vi "CLT_5PtCalStateMach.vi"(7 "Full Cfg":T4, 8 "Index In":i32, 10 "Pump Signals":T8, 11 "Cal State In":T1) -> (0 "Index Out":i32, 2 "Pump Cmds":T2, 3 "Cal State Out":T1)   [LabVIEW 2024]
doc: "The \"Run Test\" button selects between MANUAL adjustment of Set Point (SP) by the user or AUTO mode, where:\n1. Start, initial state drains until the tank is empty\n2. Filling, Auto set of SP to Max Fill Inches (or recipie)\n3. FULL Pause when full\n4. Draining Auto set of SP to 0 (or recipie)\n5. EMPTY Paue when empty\n6. Done SP set to 0."
uses:
  Control Definitions/Def_PumpSignals.ctl
  Control Definitions/Def FullCfg.ctl
  Control Definitions/Def BenchCfg.ctl
  Control Definitions/Def PumpCtlRefs.ctl
  Control Definitions/Def_PumpSpeed.ctl
  Control Definitions/Def Bench Status.ctl
  Control Definitions/Def_PumpCmds.ctl
  Control Definitions/DEF_5ptCalState.ctl
  Control Definitions/Global 2.vi
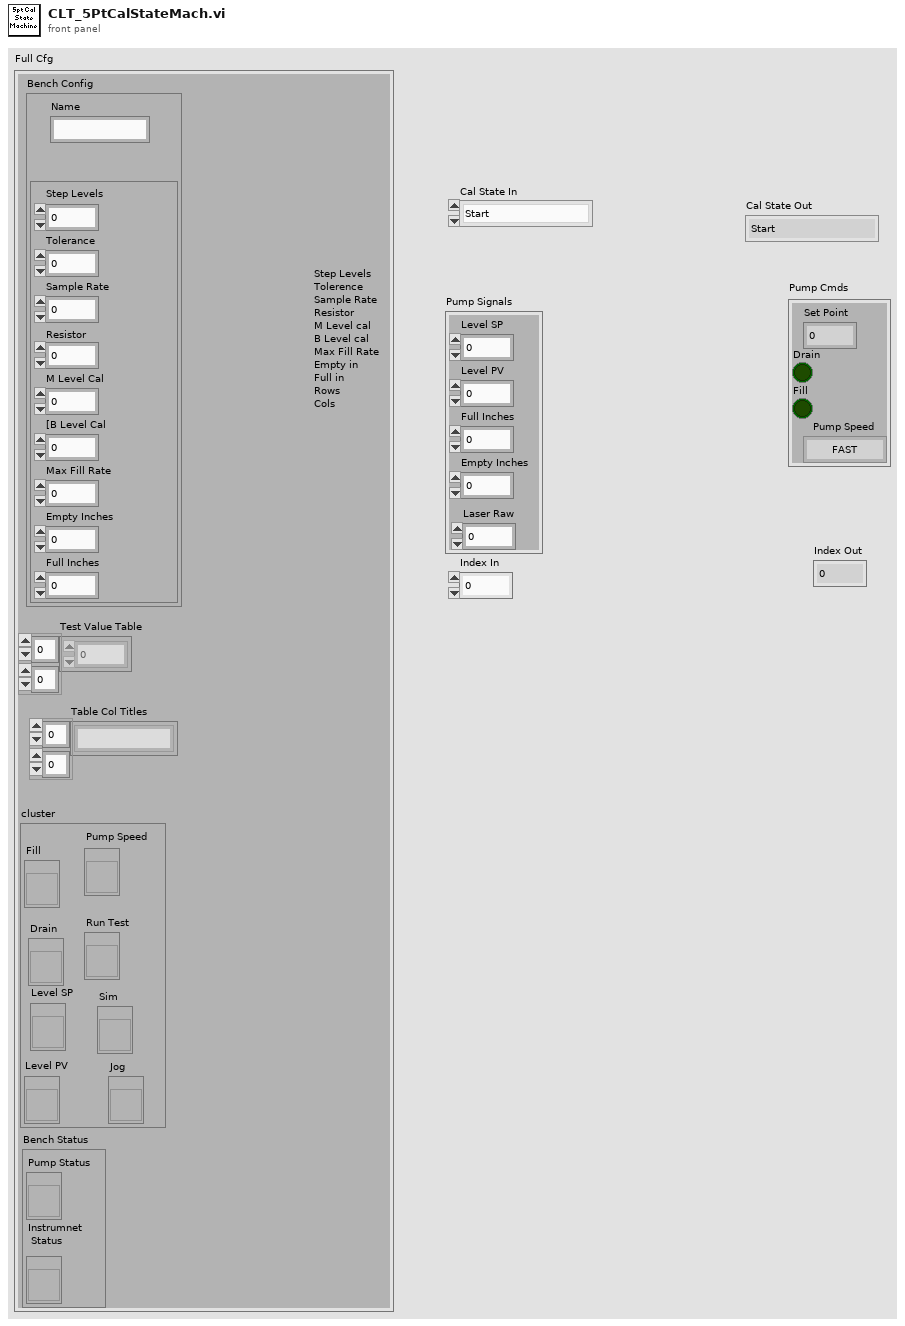
[diagram p1: front panel]
types:
  T1 = typedef "DEF_5ptCalState.ctl" = enum16{"Start", "Load Tester", "Go Auto", "Level 1", "Reveiw ", "Save", "Exit"}
  T2 = typedef "Def_PumpCmds.ctl" = cluster{"Set Point":dbl, "Drain":bool, "Fill":bool, "Pump Speed ":T3}
  T3 = typedef "Def_PumpSpeed.ctl" = enum16{"FAST", "SLOW", "CREEP", "STOP"}
  T4 = typedef "Def FullCfg.ctl" = cluster{"Bench Config":T5, "Test Value Table ":dbl[][], "Table Col Titles":string[][], "cluster":T6, "Bench Status":T7}
  T5 = typedef "Def BenchCfg.ctl" = cluster{"Name":string, cluster{"Step Levels":dbl, "Tolerance":dbl, "Sample Rate":dbl, "Resistor":dbl, "M Level Cal":dbl, "[B Level Cal":dbl, "Max Fill Rate":dbl, "Empty Inches":dbl, "Full Inches":dbl}}
  T6 = typedef "Def PumpCtlRefs.ctl" = cluster{"Fill ":refnum<vi>, "Drain":refnum<vi>, "Level PV":refnum<vi>, "Pump Speed":refnum<vi>, "Run Test":refnum<vi>, "Sim":refnum<vi>, "Jog":refnum<vi>, "Level SP":refnum<vi>}
  T7 = typedef "Def Bench Status.ctl" = cluster{"Pump Status":refnum<vi>, "Instrumnet\n Status":refnum<vi>}
  T8 = typedef "Def_PumpSignals.ctl" = cluster{"Level SP":dbl, "Level PV":dbl, "Full Inches":dbl, "Empty Inches":dbl, "Laser Raw":dbl}
  T9 = cluster{"Level SP":dbl, "X>Pos":bool, "X>Pos":bool, "Pump Speed Out":T3}
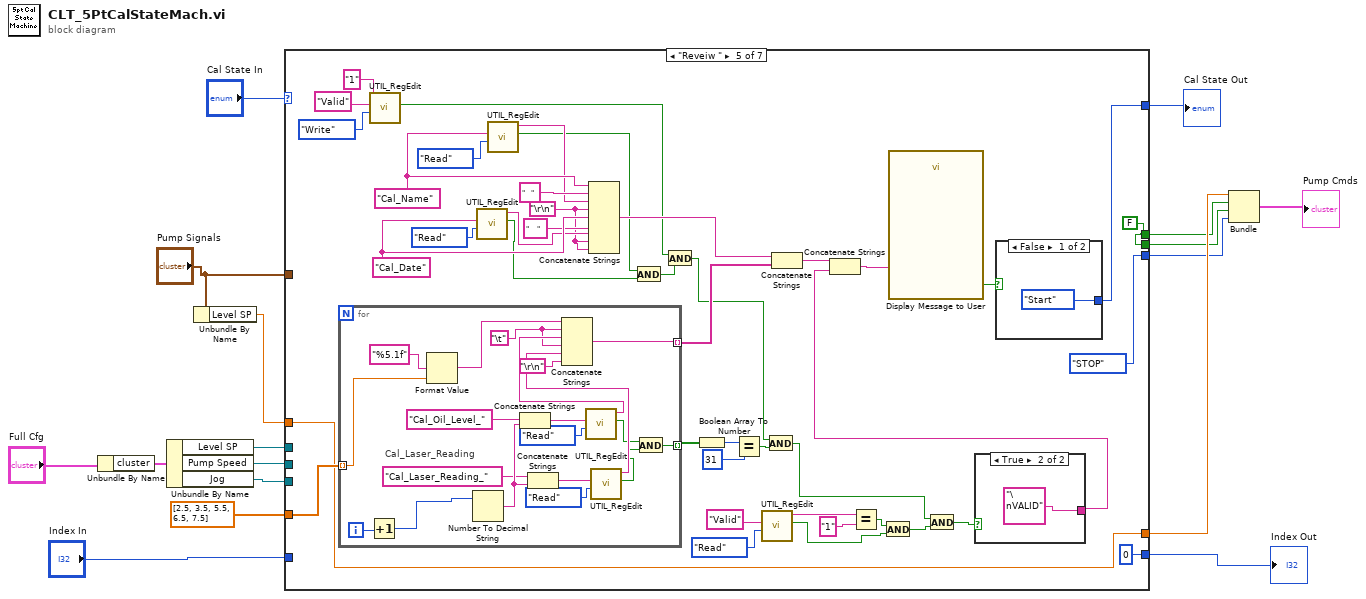
[diagram p0: block diagram]
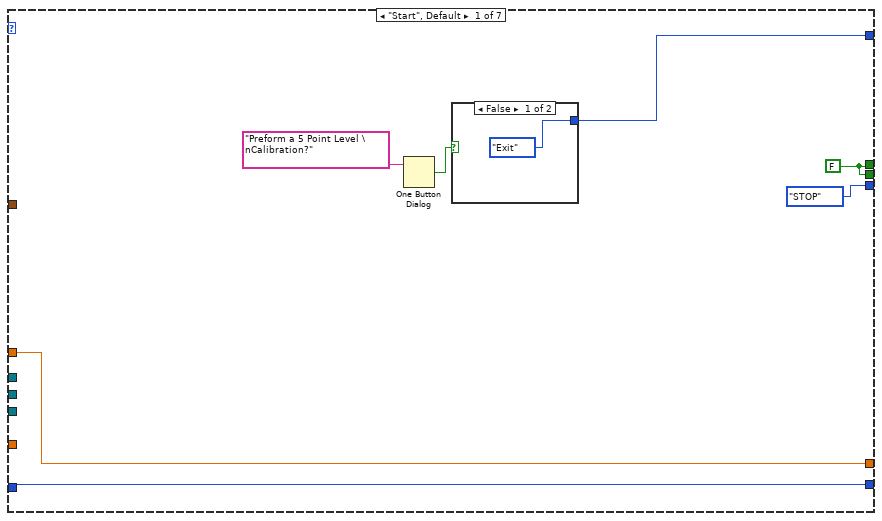
[diagram p2: hidden frame]
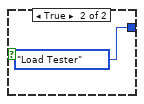
[diagram p3: hidden frame]
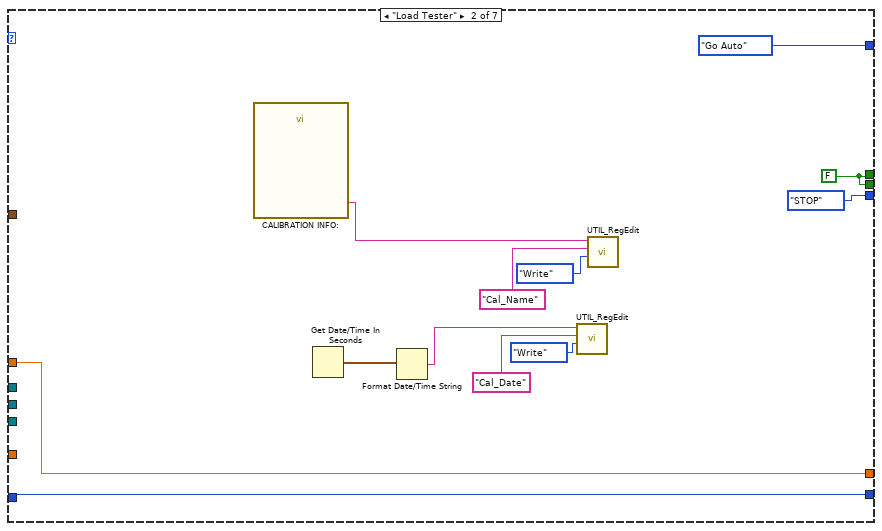
[diagram p4: hidden frame]
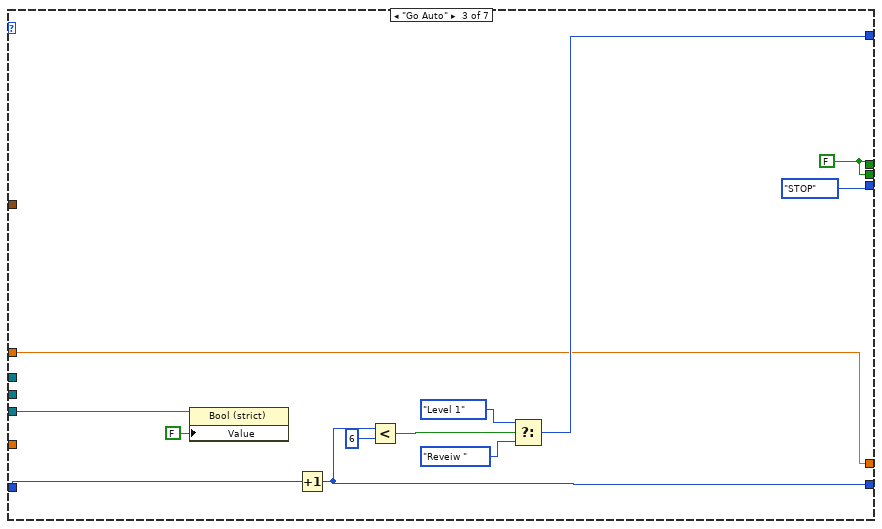
[diagram p5: hidden frame]
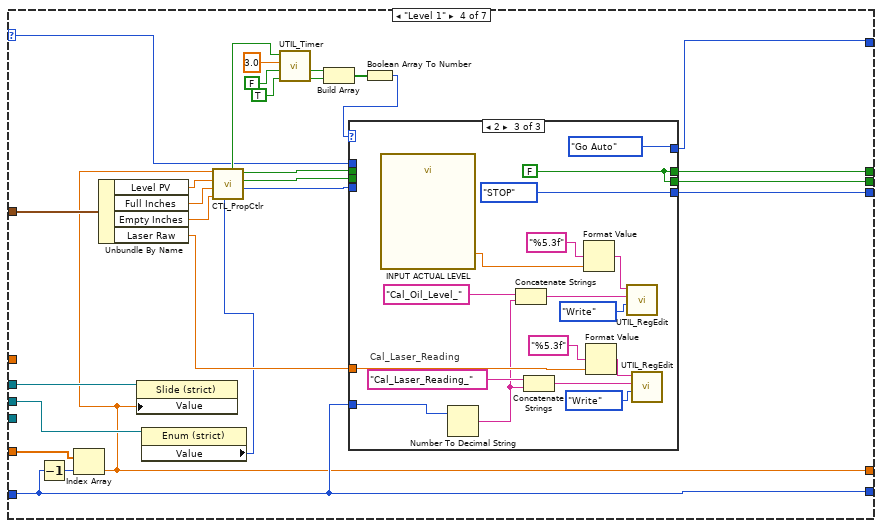
[diagram p6: hidden frame]
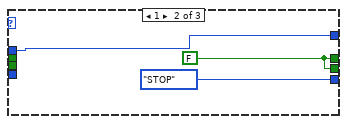
[diagram p8: hidden frame]
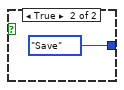
[diagram p9: hidden frame]
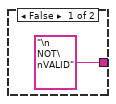
[diagram p10: hidden frame]
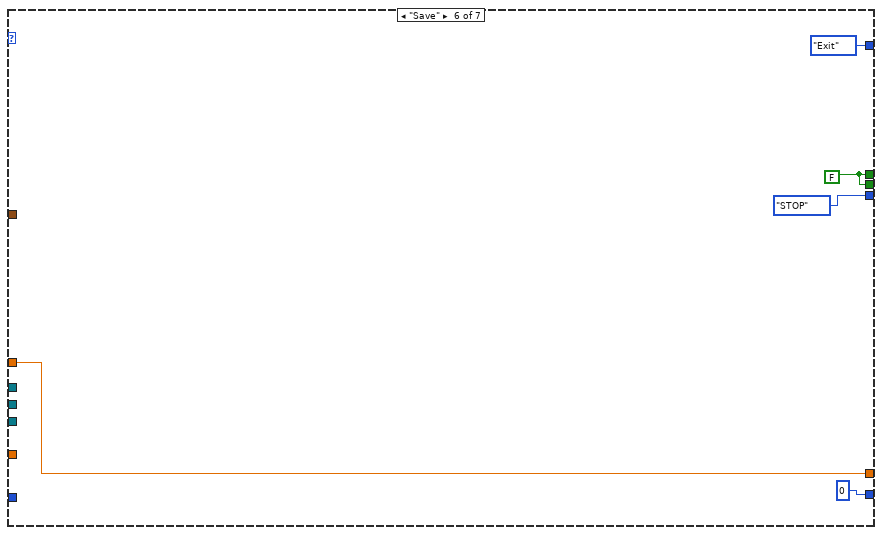
[diagram p11: hidden frame]
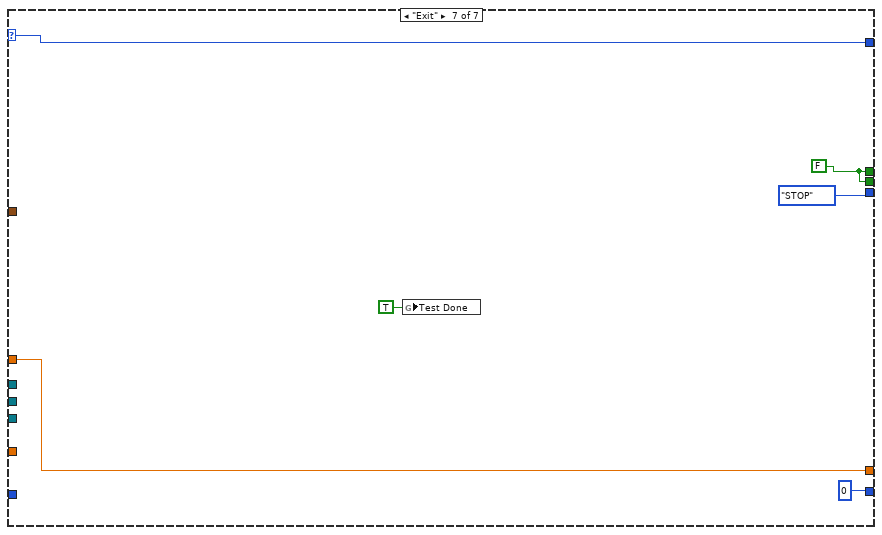
[diagram p12: hidden frame]
diagram:
  n1 = Unbundle By Name("Full Cfg") -> ("cluster"=w16:T6)
  n2 = Unbundle By Name(w16) -> ("Level SP"=w12:refnum<vi>, "Pump Speed"=w13:refnum<vi>, "Jog"=w11:refnum<vi>)
  n3 = Unbundle By Name("Pump Signals") -> ("Level SP"=w3:dbl)
  n4 = case shown="\"Reveiw \"" "Cal State In" {
    selector: "Cal State In" -> [_ _ _ w66 _ _ w175]
    tunnel: [w22 DEF_5ptCalState."Go Auto" w47 w67 w113 DEF_5ptCalState."Exit" ("Cal State In") w175] -> w14
    tunnel: "Pump Signals" -> [_ _ _ w65 _ _ _]
    tunnel: w13 -> [_ _ _ w60 _ _ _]
    tunnel: w12 -> [_ _ _ w58 _ _ _]
    tunnel: w11 -> [_ _ w50 _ _ _ _]
    tunnel: [w21 w30 w46 w55 0 0 0] -> w1
    tunnel: "Index In" -> [w21 w30 w48 w55 _ _ _]
    tunnel: dbl[] [2.5, 3.5, 5.5, 6.5, 7.5] ("Array") -> [_ _ _ w56 w135 _ _]
    tunnel: [w18 w27 w39 w51 w109 w170 w177] -> w9
    tunnel: [w20 w28 w40 w54 w111 w171 w178] -> w8
    tunnel: [w20 w28 w40 w53 w111 w171 w178] -> w7
    tunnel: [Def_PumpSpeed."STOP" ("Pump Speed Out") Def_PumpSpeed."STOP" ("Pump Speed Out") Def_PumpSpeed."STOP" ("Pump Speed Out") w52 Def_PumpSpeed."STOP" ("Pump Speed Out") Def_PumpSpeed."STOP" ("Pump Speed Out") Def_PumpSpeed."STOP" ("Pump Speed Out")] -> w6
    tunnel: w3 -> [w18 w27 w39 _ w109 w170 w177]
    frame "Start", Default {
      w20 = FALSE ("X>Pos")
      n5 = One Button Dialog(message="Preform a 5 Point Level \nCalibration?") -> (true=w23:bool)  [unwired: 1 in]
      n6 = case shown="False" w23 {
        tunnel: [DEF_5ptCalState."Exit" ("Cal State In") DEF_5ptCalState."Load Tester" ("Cal State In")] -> w22
        frame False {
        }
        frame True {
        }
      }
    }
    frame "Load Tester" {
      w28 = FALSE ("X>Pos")
      n7 = call "CALIBRATION INFO:"() -> ("Name"=w32:string)  [unwired: 17 in, 2 out]
      n8 = Get Date/Time In Seconds() -> (seconds since 1Jan1904=w37:timestamp)
      n9 = Format Date/Time String(seconds (now)=w37) -> (date/time string=w38:string)  [unwired: 2 in]
      n10 = call "UTIL_RegEdit.vi"("Mode"=enum16{"Write", "Read", "Delete"}."Write", "String Name"="Cal_Date", "String Value"=w38) -> ()  [unwired: 7 in, 2 out]
      n11 = call "UTIL_RegEdit.vi"("Mode"=enum16{"Write", "Read", "Delete"}."Write", "String Name"="Cal_Name", "String Value"=w32) -> ()  [unwired: 7 in, 2 out]
    }
    frame "Go Auto" {
      w40 = FALSE ("X>Pos")
      n12 = property class="Bool (strict)"(reference=w50, "Value"=FALSE) -> ()  [unwired: 1 in, 2 out]
      n13 = Increment(x=w48) -> (x+1=w46:i32)
      n14 = Less?(x=w46, y=6) -> (x < y?=w44:bool)
      n15 = Select(t=DEF_5ptCalState."Level 1" ("Cal State In"), s=w44, f=DEF_5ptCalState."Reveiw " ("Cal State In")) -> (s? t:f=w47:T1)
    }
    frame "Level 1" {
      n16 = Decrement(x=w55) -> (x-1=w57:i32)
      n17 = Index Array(array=w56, index=w57) -> (element=w51:dbl)
      n18 = Unbundle By Name(w65) -> ("Level PV"=w64:dbl, "Full Inches"=w63:dbl, "Empty Inches"=w62:dbl, "Laser Raw"=w61:dbl)
      n19 = property class="Slide (strict)"(reference=w58, "Value"=w51) -> ()  [unwired: 1 in, 2 out]
      n20 = property class="Enum (strict)"(reference=w60) -> ("Value"=w59:T3)  [unwired: 1 in, 2 out]
      n21 = call "CTL_PropCtlr.vi"("Pump Speed"=w59, "Empty Inches"=w62, "Full Inches"=w63, "Level PV"=w64, "Level SP"=w51) -> ("Pump Speed Out"=w68:T3, "X< Neg"=w69:bool, "X>Pos"=w71:bool, "Neg <X<Pos"=w75:bool)  [unwired: 3 in]
      n22 = call "UTIL_Timer.vi"("Auto Reset"=TRUE, "Reset"=FALSE, "Time (sec)"=3.0, "Start"=w75) -> ("Timed Out"=w73:bool, "Running"=w74:bool)  [unwired: 2 in, 4 out]
      n23 = Build Array(w74, w73) -> (w72:bool[])
      n24 = Boolean Array To Number(Boolean array=w72) -> (number=w70:u32)
      n25 = case shown="2" w70 {
        tunnel: [w82 w85 w102] -> w54
        tunnel: w71 -> [w82 _ _]
        tunnel: [w81 w85 w102] -> w53
        tunnel: w69 -> [w81 _ _]
        tunnel: [w80 Def_PumpSpeed."STOP" ("Pump Speed Out") Def_PumpSpeed."STOP" ("Pump Speed Out")] -> w52
        tunnel: w68 -> [w80 _ _]
        tunnel: [w79 w83 DEF_5ptCalState."Go Auto" ("Cal State In")] -> w67
        tunnel: w66 -> [w79 w83 _]
        tunnel: w61 -> [_ _ w96]
        tunnel: w55 -> [_ _ w92]
        frame 0, Default {
        }
        frame 1 {
          w85 = FALSE ("X>Pos")
        }
        frame 2 {
          w102 = FALSE ("X>Pos")
          # "Cal_Laser_Reading"
          n26 = call "INPUT ACTUAL LEVEL"() -> ("Level"=w93:dbl)  [unwired: 17 in, 2 out]
          n27 = Number To Decimal String(number=w92) -> (decimal integer string=w88:string)  [unwired: 1 in]
          n28 = Concatenate Strings("Cal_Oil_Level_", w88) -> (w86:string)
          n29 = Concatenate Strings("Cal_Laser_Reading_", w88) -> (w91:string)
          n30 = Format Value(format string="%5.3f", value (0)=w93) -> (output string=w94:string)  [unwired: 1 in]
          n31 = Format Value(format string="%5.3f", value (0)=w96) -> (output string=w100:string)  [unwired: 1 in]
          n32 = call "UTIL_RegEdit.vi"("Mode"=enum16{"Write", "Read", "Delete"}."Write", "String Name"=w86, "String Value"=w94) -> ()  [unwired: 7 in, 2 out]
          n33 = call "UTIL_RegEdit.vi"("Mode"=enum16{"Write", "Read", "Delete"}."Write", "String Name"=w91, "String Value"=w100) -> ()  [unwired: 7 in, 2 out]
        }
      }
    }
    frame "Reveiw " {
      w111 = FALSE ("X>Pos")
      w136 = "\r\n"
      w142 = "Cal_Name"
      w139 = "Cal_Date"
      n34 = for {
        tunnel: w135 -> [w158] mode=indexing
        tunnel: [w152] -> w133 mode=indexing
        tunnel: [w149] -> w132 mode=indexing
        i -> [w161]
        w155 = "\t"
        # "Cal_Laser_Reading"
        n35 = Increment(x=w161) -> (x+1=w160:i32)
        n36 = Format Value(format string="%5.1f", value (0)=w158) -> (output string=w157:string)  [unwired: 1 in]
        n37 = Number To Decimal String(number=w160) -> (decimal integer string=w168:string)  [unwired: 1 in]
        n38 = Concatenate Strings("Cal_Oil_Level_", w168) -> (w167:string)
        n39 = Concatenate Strings("Cal_Laser_Reading_", w168) -> (w166:string)
        n40 = call "UTIL_RegEdit.vi"("Mode"=enum16{"Write", "Read", "Delete"}."Read", "String Name"=w167) -> ("Success?"=w151:bool, "Value Read"=w156:string)  [unwired: 8 in]
        n41 = call "UTIL_RegEdit.vi"("Mode"=enum16{"Write", "Read", "Delete"}."Read", "String Name"=w166) -> ("Success?"=w150:bool, "Value Read"=w154:string)  [unwired: 8 in]
        n42 = Concatenate Strings(w157, w155, w156, w155, w154, "\r\n") -> (w152:string)
        n43 = And(x=w151, y=w150) -> (x .and. y?=w149:bool)
      }
      n44 = call "UTIL_RegEdit.vi"("Mode"=enum16{"Write", "Read", "Delete"}."Write", "String Name"="Valid", "String Value"="1") -> ("Success?"=w103:bool)  [unwired: 7 in, 1 out]
      n45 = call "UTIL_RegEdit.vi"("Mode"=enum16{"Write", "Read", "Delete"}."Read", "String Name"=w139) -> ("Success?"=w129:bool, "Value Read"=w137:string)  [unwired: 8 in]
      n46 = call "UTIL_RegEdit.vi"("Mode"=enum16{"Write", "Read", "Delete"}."Read", "String Name"=w142) -> ("Success?"=w128:bool, "Value Read"=w140:string)  [unwired: 8 in]
      n47 = Concatenate Strings(w142, "   ", w140, w136, w139, "    ", w137, w136, w136) -> (w134:string)
      n48 = And(x=w128, y=w129) -> (x .and. y?=w105:bool)
      n49 = And(x=w103, y=w105) -> (x .and. y?=w104:bool)
      n50 = Boolean Array To Number(Boolean array=w132) -> (number=w131:u32)
      n51 = Equal?(x=w131, y=u32 31) -> (x = y?=w127:bool)
      n52 = call "UTIL_RegEdit.vi"("Mode"=enum16{"Write", "Read", "Delete"}."Read", "String Name"="Valid") -> ("Success?"=w121:bool, "Value Read"=w124:string)  [unwired: 8 in]
      n53 = And(x=w104, y=w127) -> (x .and. y?=w115:bool)
      n54 = Concatenate Strings(w134, w133) -> (w119:string)
      n55 = Equal?(x=w124, y="1") -> (x = y?=w122:bool)
      n56 = And(x=w122, y=w121) -> (x .and. y?=w116:bool)
      n57 = And(x=w115, y=w116) -> (x .and. y?=w120:bool)
      n58 = case shown="True" w120 {
        tunnel: ["\n NOT\nVALID" "\nVALID"] -> w118
        frame False {
        }
        frame True {
        }
      }
      n59 = Concatenate Strings(w119, w118) -> (w117:string)
      n60 = call "Display Message to User"("Message"=w117) -> ("YES"=w114:bool)  [unwired: 9 in, 1 out]
      n61 = case shown="False" w114 {
        tunnel: [DEF_5ptCalState."Start" ("Cal State In") DEF_5ptCalState."Save" ("Cal State In")] -> w113
        frame False {
        }
        frame True {
        }
      }
    }
    frame "Save" {
      w171 = FALSE ("X>Pos")
    }
    frame "Exit" {
      w178 = FALSE ("X>Pos")
      n62 = global write "Global 2.vi" "Test Done"(TRUE ("Test Done")) -> ()
    }
  }
  "Cal State Out" <- w14
  "Index Out" <- w1
  n63 = Bundle("Level SP"=w9, "X>Pos"=w8, "X>Pos"=w7, "Pump Speed Out"=w6) -> (→"Pump Cmds":T9)  [unwired: 1 in]
